vi "List.vi"(8 "error in (no error)":errorcluster, 11 "LUnit Test Case In":refnum<class "LUnit Test Case.lvclass">) -> (0 "error out":errorcluster, 2 "List of Runnables":string[](array[string]))   [LabVIEW 2020, in "LUnit Test Case.lvclass"]
uses:
  LUnit Test Case.lvclass
  LUnit Test Case.lvclass/LUnit Test Case.ctl
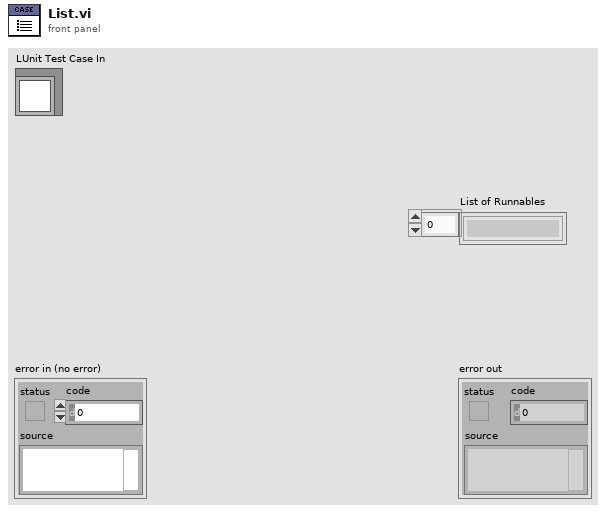
[diagram p1: front panel]
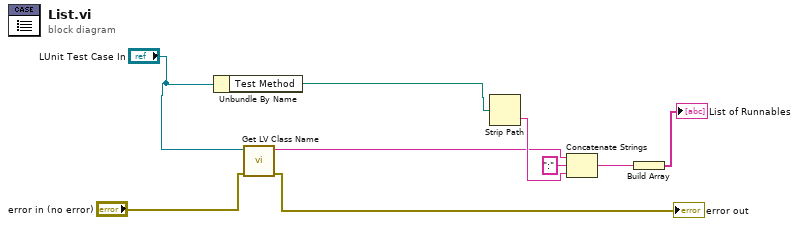
[diagram p0: block diagram]
diagram:
  n1 = Unbundle By Name("LUnit Test Case In") -> ("Test Method"=w6:path)
  n2 = call <vilib>:"Get LV Class Name.vi"("error in (no error)"="error in (no error)", "object"="LUnit Test Case In") -> ("error out"=→"error out":errorcluster, "class name"=w1:string)  [unwired: 8 in]
  n3 = Strip Path(path=w6) -> (name=w4:string)  [unwired: 1 out]
  n4 = Concatenate Strings(w1, ":" ("string"), w4) -> (w3:string)
  n5 = Build Array(w3) -> (→"List of Runnables":string[])
